vi "Stage v4.vi"() -> ()   [LabVIEW 2025]
uses:
  upper limit.ctl
  lower limit.ctl
  libximc.lvlib
panel:
  in  "Help":bool
  in  "Shift Stage Page":bool
  in  "Move to Destination Page":bool
  in  "Move Relative Page":bool
  in  "Initialize Page":bool
  in  "Tab Control":T1(tab)=enum."Shift Stage"
  out "s/n 2":u32
  out "s/n 3":u32
  out "s/n 1":u32
  in  "Controller 1":u16(ring) items=["xi-com:\\\\.\\COM3", "xi-com:\\\\.\\COM4", "xi-com:\\\\.\\COM5"]
  in  "Controller 2":u16(ring) items=["xi-com:\\\\.\\COM3", "xi-com:\\\\.\\COM4", "xi-com:\\\\.\\COM5"]
  in  "Controller 3":u16(ring) items=["xi-com:\\\\.\\COM3", "xi-com:\\\\.\\COM4", "xi-com:\\\\.\\COM5"]
  in  "Move To Destination":bool
  in  "Destination X":dbl format="%#.3f"
  in  "Destination Z":dbl format="%#.3f"
  in  "Destination Y":dbl format="%#.3f"
  in  "Update Position":bool
  in  "Paste Positions":bool
  in  "Shift X":dbl format="%#.3f"
  in  "Shift Z":dbl format="%#.3f"
  in  "Shift Y":dbl format="%#.3f"
  in  "Move Relative":bool
  in  "shift stage":bool
  in  "Shift Amount (mm)":dbl format="%#.3f"
  in  "Copy Positions":bool
  in  "Zero":bool
  in  "Go Home":bool
  in  "Exit":bool
  out "Cursor Z":dbl format="%.3f"
  out "Cursor Y":dbl format="%.3f"
  out "Cursor X":dbl format="%.3f"
  # "Controller IDs"
  # "Serial Numbers"
  # "Controller Y"
  # "Controller X"
  # "Controller Z"
  # "If serial numbers are 0, click the help button!"
  # "NOTE: Units of all positions are in mm."
  # "Stage not moving:"
  # "Check if the serial numbers are zero. If so, close this app and load the controllers in order (1, 2, then 3) in XILab. Close XILab and open this app. and controllers should load correctly."
  # "Controllers not found in XILab:"
  # "Unplug and replug USBs connecting the motors to the computer, then follow previous instructions."
  # "If you have any other questions, feel free to reach out to Erykah at erykahfoss@u.boisestate.edu"
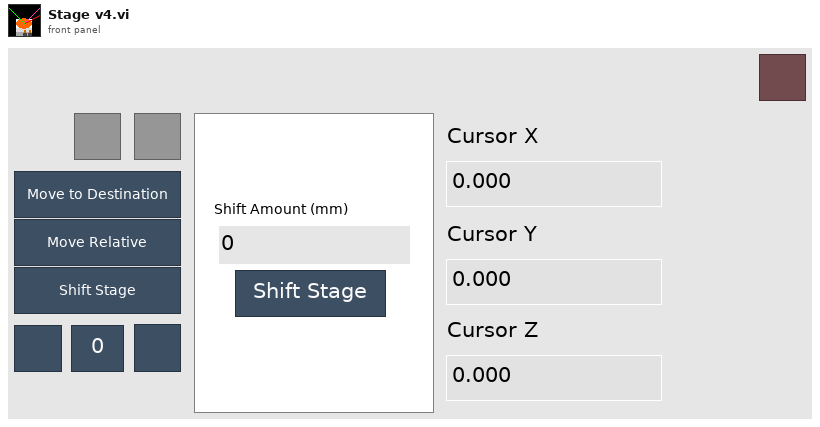
[diagram p1: front panel]
types:
  T1 = enum32{"Initialize", "Help", "Move to Destination", "Move Relative", "Shift Stage"}
  T2 = enum16{"Initialize", "Help", "Move to Destination", "Move Relative", "Shift Stage"}
  T3 = enum32{"invalid app kind", "Development System", "Run Time System", "Student Edition", "Embedded LabVIEW", "Evaluation", "Custom"}
  T4 = cluster{"Number of controllers":i32, "Controllers' names":string[], "variant":variant, "quit":bool, "IDs":i32[]}
  T5 = typedef "eventvkey.ctl" = enum16{"ASCII", "Enter", "Return", "Shift", "Ctrl", "Alt", "Cmd", "Opt", "Caps", "NumLock", "Clear", "Break", "Up", "Down", "Left", "Right", "Insert", "Delete", "Home", "End", "PageUp", "PageDown", "Escape", "Help", "Pause", "ScrollLock", "F1", "F2", "F3", "F4", "F5", "F6", "F7", "F8", "F9", "F10", "F11", "F12", "F13", "F14", "F15", "F16", "F17", "F18", "F19", "F20", "F21", "F22", "F23", "F24", "Play", "VolumeUp", "VolumeDown", "Mute", "Two Byte Char"}
  T6 = typedef "lower limit.ctl" = i32
  T7 = typedef "upper limit.ctl" = i32
  T8 = cluster{"MoveSts":u32, "MvCmdSts":u32, "PWRSts":u32, "EncSts":u32, "WindSts":u32, "CurPosition":i32, "uCurPosition":i32, "@dummy control@":i8, "@dummy control@":i8, "@dummy control@":i8, "@dummy control@":i8, "EncPosition":i64, "CurSpeed":i32, "uCurSpeed":i32, "Ipwr":i32, "Upwr":i32, "Iusb":i32, "Uusb":i32, "CurT":i32, "Flags":u32, "GPIOFlags":u32, "CmdBufFreeSpace":u32}
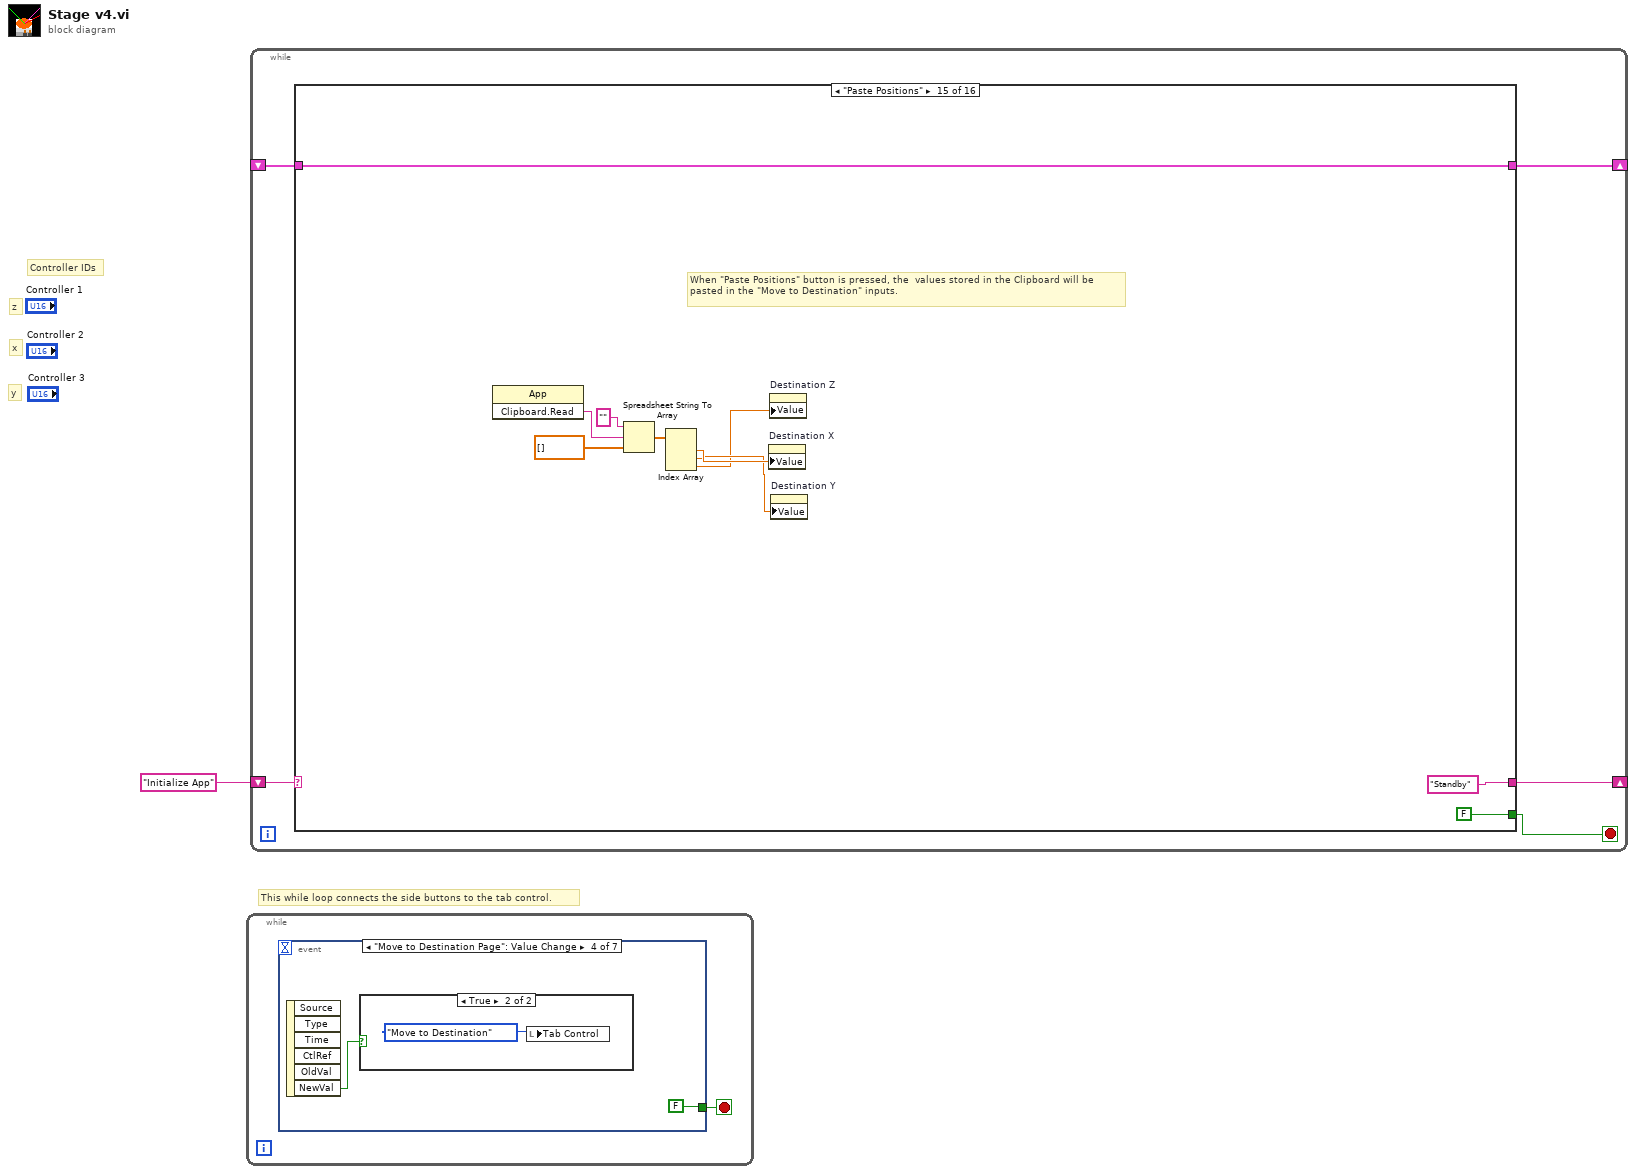
[diagram p0: block diagram]
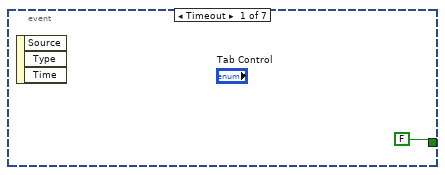
[diagram p2: hidden frame]
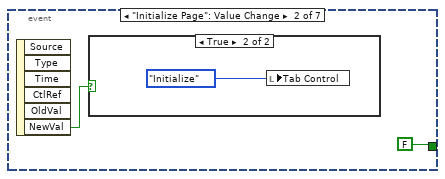
[diagram p3: hidden frame]
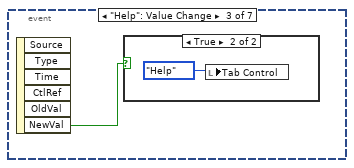
[diagram p5: hidden frame]
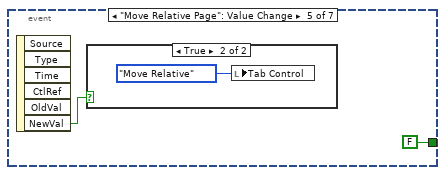
[diagram p8: hidden frame]
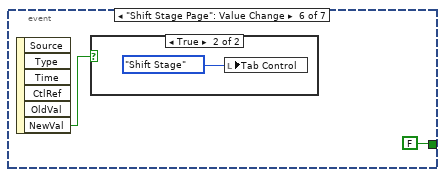
[diagram p10: hidden frame]
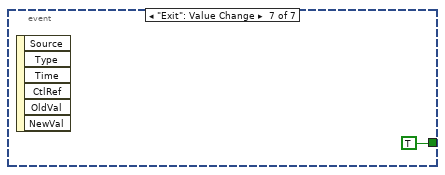
[diagram p12: hidden frame]
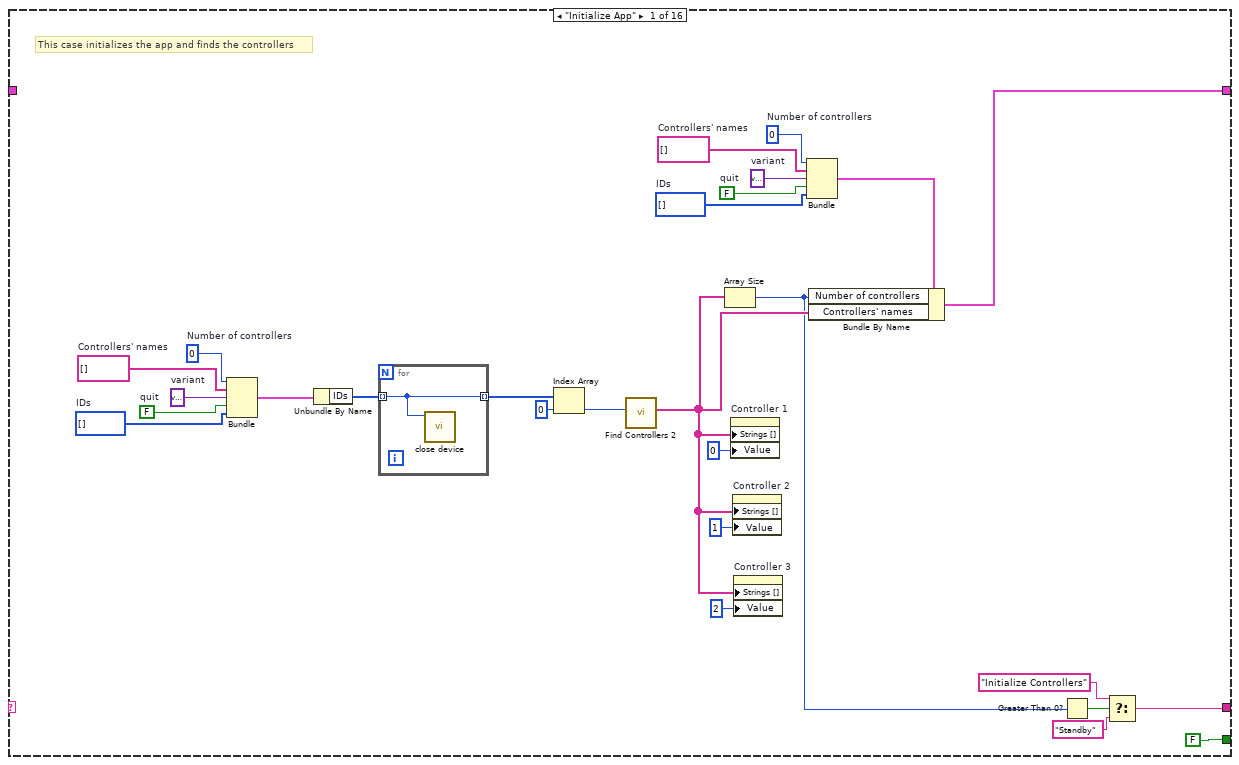
[diagram p13: hidden frame]
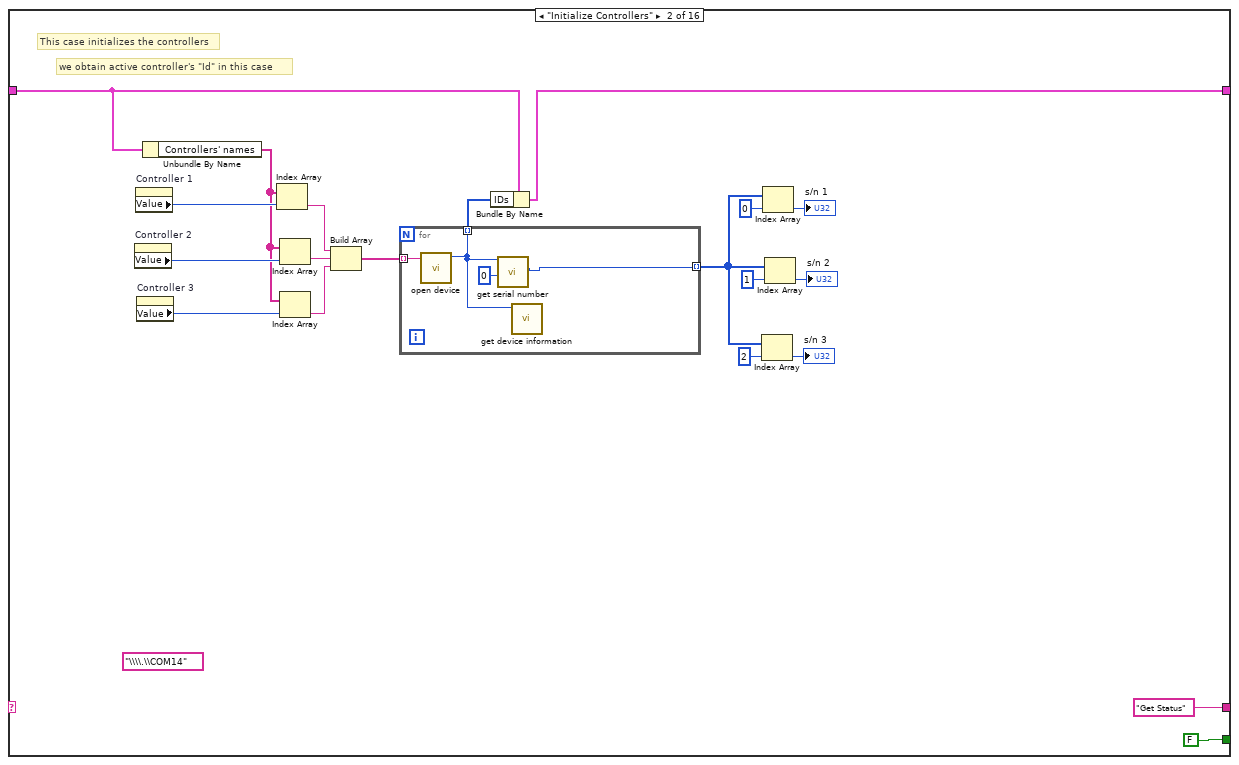
[diagram p14: hidden frame]
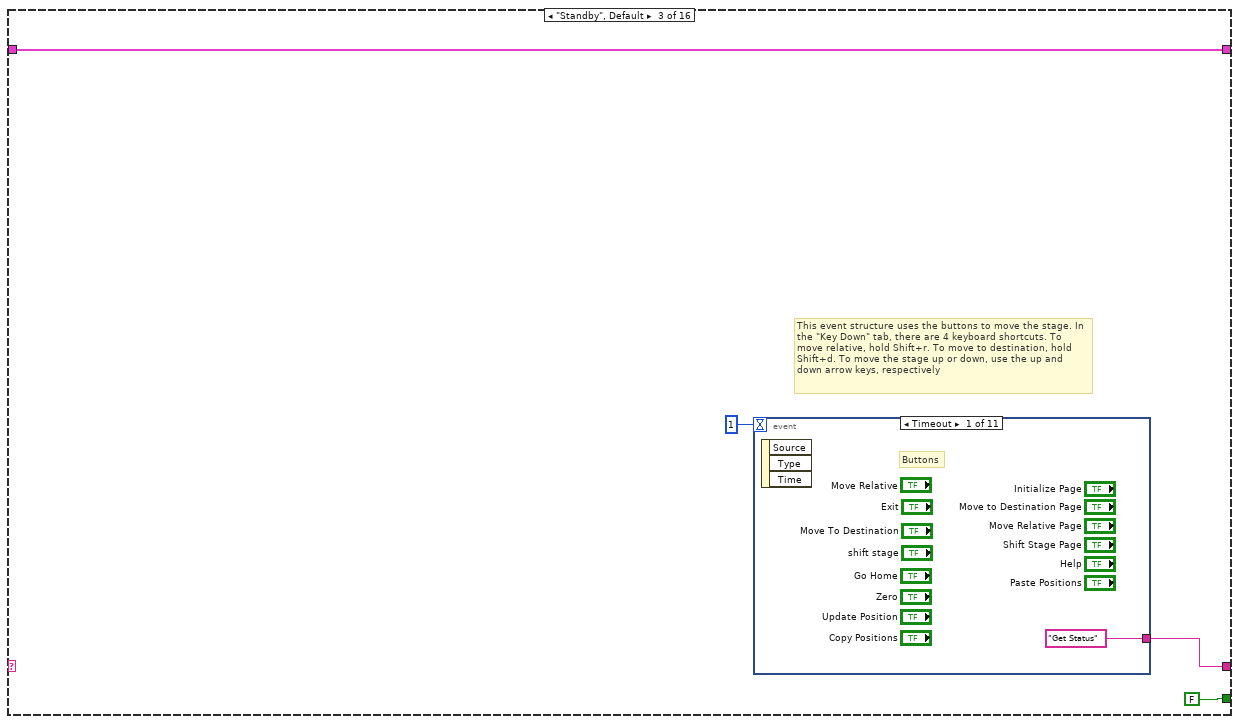
[diagram p15: hidden frame]
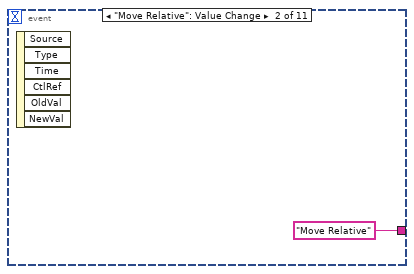
[diagram p16: hidden frame]
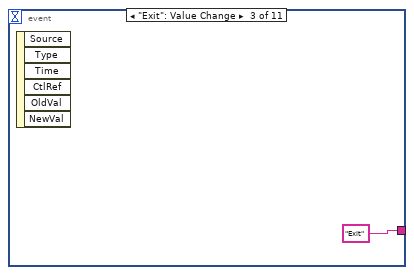
[diagram p17: hidden frame]
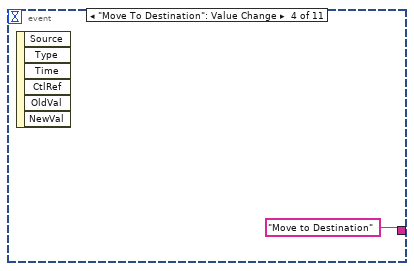
[diagram p18: hidden frame]
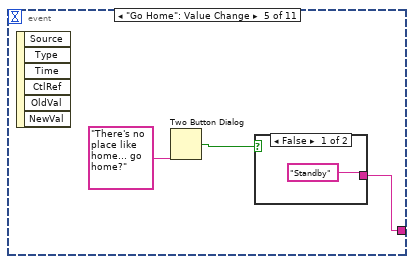
[diagram p19: hidden frame]
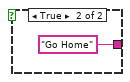
[diagram p20: hidden frame]
diagram:
  # "y"
  # "x"
  # "z"
  # "This while loop connects the side buttons to the tab control."
  # "Controller IDs"
  n1 = while {
    stop <- w2 stop-if-true
    n2 = event shown="[3] \"Move to Destination Page\": Value Change" {
      selector: _ -> [_ _ _ _ _ _ _]
      dyn-events: _ -> [_ _ _ _ _ _ _]
      timeout: _ -> [_ _ _ _ _ _ _]
      tunnel: [FALSE FALSE _ FALSE FALSE FALSE TRUE] -> w2
      event Timeout {
        n3 = event-data() -> ()  [unwired: 1 in, 3 out]
      }
      event "Initialize Page": Value Change {
        n4 = event-data() -> ("NewVal"=w4:bool)  [unwired: 1 in, 5 out]
        n5 = case shown="True" w4 {
          frame False {
          }
          frame True {
            n6 = local write "Tab Control"(T2."Initialize") -> ()
          }
        }
      }
      event "Help": Value Change {
        n7 = event-data() -> ("NewVal"=w7:bool)  [unwired: 1 in, 5 out]
        n8 = case shown="True" w7 {
          frame False {
          }
          frame True {
            n9 = local write "Tab Control"(T2."Help") -> ()
          }
        }
      }
      event "Move to Destination Page": Value Change {
        n10 = event-data() -> ("NewVal"=w9:bool)  [unwired: 1 in, 5 out]
        n11 = case shown="True" w9 {
          frame False {
          }
          frame True {
            n12 = local write "Tab Control"(T2."Move to Destination") -> ()
          }
        }
      }
      event "Move Relative Page": Value Change {
        n13 = event-data() -> ("NewVal"=w12:bool)  [unwired: 1 in, 5 out]
        n14 = case shown="True" w12 {
          frame False {
          }
          frame True {
            n15 = local write "Tab Control"(T2."Move Relative") -> ()
          }
        }
      }
      event "Shift Stage Page": Value Change {
        n16 = event-data() -> ("NewVal"=w15:bool)  [unwired: 1 in, 5 out]
        n17 = case shown="True" w15 {
          frame False {
          }
          frame True {
            n18 = local write "Tab Control"(T2."Shift Stage") -> ()
          }
        }
      }
      event "Exit": Value Change {
        n19 = event-data() -> ()  [unwired: 1 in, 6 out]
      }
    }
  }
  n20 = while {
    shift-right: [w22] -> _
    shift-left: _ -> [w23]
    shift-right: [w21] -> _
    shift-left: "Initialize App" -> [w20]
    stop <- w19 stop-if-true
    n21 = case shown="\"Paste Positions\"" w20 {
      tunnel: [w44 w61 w79 w125 w175 w240 w292 w349 w411 w460 w465 w470 w482 w504 w514 w522] -> w22
      tunnel: w23 -> [_ w62 w79 w125 w175 w239 w292 w349 w411 w460 w465 w470 w482 w504 w514 w522]
      tunnel: [w25 "Get Status" w77 w138 w174 w238 w291 w348 w410 "Standby" "Standby" "Standby" "Standby" "Standby" "Standby" "Standby"] -> w21
      tunnel: [FALSE ("quit") FALSE ("quit") FALSE ("quit") w127 FALSE ("quit") FALSE ("quit") FALSE FALSE FALSE FALSE FALSE FALSE FALSE FALSE FALSE TRUE ("quit")] -> w19
      frame "Initialize App" {
        w31 = i32[] []  # IDs
        w32 = FALSE  # quit
        w33 = variant  # variant
        w34 = string[] []  # Controllers' names
        w35 = 0  # Number of controllers
        w46 = i32[] []  # IDs
        w47 = FALSE  # quit
        w48 = variant  # variant
        w49 = string[] []  # Controllers' names
        w50 = 0  # Number of controllers
        # "This case initializes the app and finds the controllers"
        n22 = Bundle("Number of controllers"=w35, "Controllers' names"=w34, "variant"=w33, "quit"=w32, "IDs"=w31) -> (w30:T4)  [unwired: 1 in]
        n23 = Unbundle By Name(w30) -> ("IDs"=w37:i32[])
        n24 = for {
          tunnel: w37 -> [w51] mode=indexing
          tunnel: [w51] -> w36 mode=indexing
          n25 = call "close device.vi"("id"=w51) -> ()  [unwired: 8 in, 3 out]
        }
        n26 = Index Array(array=w36, index=0) -> (element=w42:i32)
        n27 = call "Find Controllers 2.vi"("Numeric"=w42) -> ("Names"=w38:string[])  [unwired: 9 in, 1 out]
        n28 = Array Size(array=w38) -> (size(s)=w28:i32)
        n29 = property on="Controller 1" class="Ring (strict)"("Strings []"=w38, "Value"=0) -> ()  [unwired: 2 in, 2 out]
        n30 = property on="Controller 2" class="Ring (strict)"("Strings []"=w38, "Value"=1) -> ()  [unwired: 2 in, 2 out]
        n31 = property on="Controller 3" class="Ring (strict)"("Strings []"=w38, "Value"=2 ("Controller 3")) -> ()  [unwired: 2 in, 2 out]
        n32 = Bundle("Number of controllers"=w50, "Controllers' names"=w49, "variant"=w48, "quit"=w47, "IDs"=w46) -> (w45:T4)  [unwired: 1 in]
        n33 = Bundle By Name(cluster=w45, "Number of controllers"=w28, "Controllers' names"=w38) -> (w44:T4)
        n34 = Greater Than 0?(x=w28) -> (x > 0?=w29:bool)
        n35 = Select(t="Initialize Controllers", s=w29, f="Standby") -> (s? t:f=w25:string)
      }
      frame "Initialize Controllers" {
        (unwired) "\\\\.\\COM14" ("name")
        # "we obtain active controller's \"Id\" in this case"
        # "This case initializes the controllers"
        n36 = property on="Controller 2" class="Ring (strict)"() -> ("Value"=w70:u16)  [unwired: 2 in, 2 out]
        n37 = property on="Controller 1" class="Ring (strict)"() -> ("Value"=w71:u16)  [unwired: 2 in, 2 out]
        n38 = property on="Controller 3" class="Ring (strict)"() -> ("Value"=w69:u16)  [unwired: 2 in, 2 out]
        n39 = Unbundle By Name(w62) -> ("Controllers' names"=w65:string[])
        n40 = Index Array(array=w65, index=w71) -> (element=w66:string)
        n41 = Index Array(array=w65, index=w70) -> (element=w67:string)
        n42 = Index Array(array=w65, index=w69) -> (element=w68:string)
        n43 = Build Array(w66, w67, w68) -> (w64:string[])
        n44 = for {
          tunnel: w64 -> [w75] mode=indexing
          tunnel: [w73] -> w63 mode=indexing
          tunnel: [w72] -> w54 mode=indexing
          n45 = call "open device.vi"("uri"=w75) -> ("function return"=w73:i32)  [unwired: 9 in, 1 out]
          n46 = call "get serial number.vi"("SerialNumber"=0, "id"=w73) -> ("SerialNumber out"=w72:u32)  [unwired: 7 in, 2 out]
          n47 = call "get device information.vi"("id"=w73) -> ()  [unwired: 8 in, 3 out]
        }
        n48 = Bundle By Name(cluster=w62, "IDs"=w63) -> (w61:T4)
        n49 = Index Array(array=w54, index=u32 2 ("serial")) -> (element=→"s/n 3":u32)
        n50 = Index Array(array=w54, index=u32 0 ("serial")) -> (element=→"s/n 1":u32)
        n51 = Index Array(array=w54, index=u32 1 ("serial")) -> (element=→"s/n 2":u32)
      }
      frame "Standby", Default {
        # "This event structure uses the buttons to move the stage. In the \"Key Down\" tab, there are 4 keyboard shortcuts. To move relative, hold Shift+r. To move to destination, hold Shift+d. To move the stage up or down, use the up and down arrow keys, respectively"
        n52 = event shown="[0] Timeout" {
          selector: _ -> [_ _ _ _ _ _ _ _ _ _ _]
          dyn-events: _ -> [_ _ _ _ _ _ _ _ _ _ _]
          timeout: 1 -> [_ _ _ _ _ _ _ _ _ _ _]
          tunnel: ["Get Status" "Move Relative" "Exit" "Move to Destination" w86 w91 "Shift Stage" "Update Position" "Copy Positions" "Paste Positions" w100] -> w77
          event Timeout {
            # "Buttons"
            n53 = event-data() -> ()  [unwired: 1 in, 3 out]
          }
          event "Move Relative": Value Change {
            n54 = event-data() -> ()  [unwired: 1 in, 6 out]
          }
          event "Exit": Value Change {
            n55 = event-data() -> ()  [unwired: 1 in, 6 out]
          }
          event "Move To Destination": Value Change {
            n56 = event-data() -> ()  [unwired: 1 in, 6 out]
          }
          event "Go Home": Value Change {
            n57 = event-data() -> ()  [unwired: 1 in, 6 out]
            n58 = Two Button Dialog(message="There's no place like home... go home?") -> (T button?=w85:bool)  [unwired: 2 in]
            n59 = case shown="False" w85 {
              tunnel: ["Standby" "Go Home"] -> w86
              frame False {
              }
              frame True {
              }
            }
          }
          event "Zero": Value Change {
            n60 = event-data() -> ()  [unwired: 1 in, 6 out]
            n61 = Two Button Dialog(message="Zero stage?") -> (T button?=w89:bool)  [unwired: 2 in]
            n62 = case shown="False" w89 {
              tunnel: ["Standby" "Zero"] -> w91
              frame False {
              }
              frame True {
              }
            }
          }
          event "shift stage": Value Change {
            n63 = event-data() -> ()  [unwired: 1 in, 6 out]
          }
          event "Update Position": Value Change {
            n64 = event-data() -> ()  [unwired: 1 in, 6 out]
          }
          event "Copy Positions": Value Change {
            n65 = event-data() -> ()  [unwired: 1 in, 6 out]
          }
          event "Paste Positions": Value Change {
            n66 = event-data() -> ()  [unwired: 1 in, 6 out]
          }
          event Key Down {
            n67 = event-data() -> ("Char"=w99:i16, "VKey"=w98:T5)  [unwired: 1 in]
            n68 = case shown="0, Default" w99 {
              tunnel: [w101 "Move Relative" "Move to Destination" "Standby" "Standby"] -> w100
              tunnel: w98 -> [w102 _ _ _ _]
              frame 0, Default {
                n69 = case shown="\"ASCII\", Default" w102 {
                  tunnel: ["Get Status" "Shift Up" "Shift Down"] -> w101
                  frame "ASCII", Default {
                  }
                  frame "Up" {
                  }
                  frame "Down" {
                  }
                }
              }
              frame 82 {
              }
              frame 68 {
              }
              frame 102 {
                n70 = call <vilib>:"Application Directory.vi"() -> ("Application Directory"=w111:path)
                n71 = String To Path(string="f.wav") -> (path=w109:path)
                n72 = Build Path(base path=w111, name or relative path=w109) -> (appended path=w108:path)
                n73 = call <vilib>:"Play Sound File.vi"("path"=w108) -> ()  [unwired: 9 in, 2 out]
              }
              frame 108 {
                n74 = call <vilib>:"Application Directory.vi"() -> ("Application Directory"=w116:path)
                n75 = String To Path(string="l.wav") -> (path=w114:path)
                n76 = Build Path(base path=w116, name or relative path=w114) -> (appended path=w113:path)
                n77 = call <vilib>:"Play Sound File.vi"("path"=w113) -> ()  [unwired: 9 in, 2 out]
              }
            }
          }
        }
      }
      frame "Get Status" {
        w123 = 8.3e-05
        w126 = T6 -600
        w128 = T7 156626
        # "step to mm"
        # "cursor 3"
        # "cursor 2"
        # "cursor 1"
        # "lower limit"
        # "upper limit"
        # "Note: The upper limit comes from a calculation. The motor upper limit is 13 mm, and a step size is 0.083 um (https://www.standa.lt/products/catalog/motorised_positioners?item=315). The conversion is then 13 mm = 156,626 steps. Assuming that the motors are zeroed at the lowest height, the lower limit would be 0 mm = 0 steps and the upper limit would be 13 mm = 156,626 steps.\n\nMotors can't be zeroed in this LabVIEW program... this would be a good thing to include."
        # "These \"OR\" statements should check if any of the motors are at or above their upper limits or at or below thier lower limits."
        n78 = Unbundle By Name(w125) -> ("IDs"=w147:i32[])
        n79 = for {
          tunnel: [w161] -> w145 mode=indexing
          tunnel: w147 -> [w160] mode=indexing
          tunnel: [w159] -> w146 mode=indexing
          n80 = call "get status.vi"("id"=w160) -> ("status out"=w158:T8, "function return"=w159:i32)  [unwired: 8 in, 1 out]
          n81 = Unbundle By Name(w158) -> ("CurPosition"=w161:i32)
        }
        n82 = Greater Or Equal To 0?(x=w146) -> (x >= 0?=w141:bool[])
        n83 = And Array Elements(Boolean array=w141) -> ()  [unwired: 1 out]
        n84 = Index Array(array=w145, index #1=0 ("index"), index #2=1 ("index"), index #3=2 ("index")) -> (element #1=w124:i32, element #2=w122:i32, element #3=w121:i32)
        n85 = Less?(x=w124, y=w126) -> (x < y?=w139:bool)
        n86 = Greater Or Equal?(x=w124, y=w128) -> (x >= y?=w140:bool)
        n87 = Multiply(x=w123, y=w124) -> (x*y=→"Cursor Z":dbl)
        n88 = Multiply(x=w123, y=w122) -> (x*y=→"Cursor X":dbl)
        n89 = Multiply(x=w123, y=w121) -> (x*y=→"Cursor Y":dbl)
        n90 = Or(x=w140, y=w139) -> (x .or. y?=w133:bool)
        n91 = Greater Or Equal?(x=w122, y=w128) -> (x >= y?=w137:bool)
        n92 = Less?(x=w122, y=w126) -> (x < y?=w136:bool)
        n93 = Or(x=w137, y=w136) -> (x .or. y?=w132:bool)
        n94 = Greater Or Equal?(x=w121, y=w128) -> (x >= y?=w135:bool)
        n95 = Less?(x=w121, y=w126) -> (x < y?=w134:bool)
        n96 = Or(x=w135, y=w134) -> (x .or. y?=w131:bool)
        n97 = Build Array(w133, w132, w131) -> (w130:bool[])
        n98 = Or Array Elements(Boolean array=w130) -> (logical OR=w129:bool)
        n99 = case shown="False" w129 {
          tunnel: ["Standby" "Stop Motion"] -> w138
          tunnel: [FALSE w155] -> w127
          frame False {
          }
          frame True {
            # "If any of them move past the limits, the program will stop. You won't be able to use this LabVIEW program until the height is fixed in XILab."
            n100 = call <vilib>:"Application Directory.vi"() -> ("Application Directory"=w154:path)
            n101 = String To Path(string="l.wav") -> (path=w152:path)
            n102 = Build Path(base path=w154, name or relative path=w152) -> (appended path=w151:path)
            n103 = call <vilib>:"Sound File Read Simple.vi"("path"=w151) -> ("path out"=w150:path)  [unwired: 7 in, 3 out]
            n104 = call <vilib>:"Play Sound File.vi"("path"=w150) -> ()  [unwired: 9 in, 2 out]
            n105 = One Button Dialog(message="You've gone too far this time...\nPlease check the height of the stage and move it back to a normal height using XILab <3") -> (true=w155:bool)  [unwired: 1 in]
          }
        }
      }
      frame "Move Relative" {
        w171 = 8.3e-05
        w172 = T7 156626
        w173 = -1
        # "mm to step"
        # "in mm"
        # "cursor 3"
        # "cursor 2"
        # "cursor 1"
        # "lower limit"
        # "upper limit"
        n106 = Unbundle By Name(w175) -> ("IDs"=w199:i32[])
        n107 = for {
          tunnel: [w225] -> w197 mode=indexing
          tunnel: w199 -> [w224] mode=indexing
          tunnel: [w223] -> w198 mode=indexing
          n108 = call "get status.vi"("id"=w224) -> ("status out"=w222:T8, "function return"=w223:i32)  [unwired: 8 in, 1 out]
          n109 = Unbundle By Name(w222) -> ("CurPosition"=w225:i32)
        }
        n110 = Greater Or Equal To 0?(x=w198) -> (x >= 0?=w193:bool[])
        n111 = And Array Elements(Boolean array=w193) -> ()  [unwired: 1 out]
        n112 = Index Array(array=w197, index #1=0 ("index"), index #2=1 ("index"), index #3=2 ("index")) -> (element #1=w181:i32, element #2=w180:i32, element #3=w179:i32)
        n113 = Divide(x="Shift Y", y=w171) -> (x/y=w167:dbl)
        n114 = Divide(x="Shift Z", y=w171) -> (x/y=w165:dbl)
        n115 = Divide(x="Shift X", y=w171) -> (x/y=w163:dbl)
        n116 = To Long Integer(number=w167) -> (32bit integer=w166:i32)
        n117 = To Long Integer(number=w165) -> (32bit integer=w164:i32)
        n118 = Add(x=w166, y=w181) -> (x+y=w178:i32)
        n119 = Add(x=w164, y=w180) -> (x+y=w176:i32)
        n120 = To Long Integer(number=w163) -> (32bit integer=w162:i32)
        n121 = Add(x=w162, y=w179) -> (x+y=w177:i32)
        n122 = Less Or Equal?(x=w178, y=w173) -> (x <= y?=w191:bool)
        n123 = Greater Or Equal?(x=w177, y=w172) -> (x >= y?=w188:bool)
        n124 = Greater Or Equal?(x=w178, y=w172) -> (x >= y?=w192:bool)
        n125 = Greater Or Equal?(x=w176, y=w172) -> (x >= y?=w190:bool)
        n126 = Less Or Equal?(x=w176, y=w173) -> (x <= y?=w189:bool)
        n127 = Less Or Equal?(x=w177, y=w173) -> (x <= y?=w187:bool)
        n128 = Or(x=w188, y=w187) -> (x .or. y?=w184:bool)
        n129 = Or(x=w190, y=w189) -> (x .or. y?=w185:bool)
        n130 = Or(x=w192, y=w191) -> (x .or. y?=w186:bool)
        n131 = Build Array(w186, w185, w184) -> (w183:bool[])
        n132 = Or Array Elements(Boolean array=w183) -> (logical OR=w182:bool)
        n133 = case shown="False" w182 {
          tunnel: ["Standby" "Stop Motion"] -> w174
          tunnel: w175 -> [w211 w219]
          tunnel: [w209 w219] -> _
          tunnel: w166 -> [w203 _]
          tunnel: w164 -> [w202 _]
          tunnel: w162 -> [w201 _]
          frame False {
            n134 = Bundle(w202, w201, w203) -> (w210:cluster{i32, i32, i32})  [unwired: 1 in]
            n135 = Bundle By Name(cluster=w211, "variant"=w210) -> (w209:T4)
            n136 = Unbundle By Name(w209) -> ("IDs"=w204:i32[], "variant"=w206:variant)
            n137 = Variant To Data(type=cluster{u32, u32, u32} {0, 0, 0}, Variant=w206) -> (data=w207:cluster{u32, u32, u32})  [unwired: 1 in, 1 out]
            n138 = Cluster To Array(cluster=w207) -> (array=w208:u32[])
            n139 = for {
              tunnel: w208 -> [w213] mode=indexing
              tunnel: w204 -> [w214] mode=indexing
              n140 = call "command movr.vi"("DeltaPosition"=w213, "id"=w214) -> ()  [unwired: 8 in, 2 out]
            }
          }
          frame True {
            # "If any of them move past the limits, the motors won't move."
            n141 = call <vilib>:"Application Directory.vi"() -> ("Application Directory"=w218:path)
            n142 = String To Path(string="l.wav") -> (path=w216:path)
            n143 = Build Path(base path=w218, name or relative path=w216) -> (appended path=w215:path)
            n144 = One Button Dialog(message="You've gone too far this time...\nPlease ensure the step size does not go past the limits <3") -> ()  [unwired: 1 in, 1 out]
            n145 = call <vilib>:"Play Sound File.vi"("path"=w215) -> ()  [unwired: 9 in, 2 out]
          }
        }
      }
      frame "Move to Destination" {
        w232 = 8.3e-05
        w236 = T7 156626
        w237 = -1
        # "mm to step"
        # "cursor 3"
        # "cursor 2"
        # "cursor 1"
        # "lower limit"
        # "upper limit"
        n146 = Unbundle By Name(w239) -> ("IDs"=w258:i32[])
        n147 = for {
          tunnel: [w284] -> w256 mode=indexing
          tunnel: w258 -> [w283] mode=indexing
          tunnel: [w282] -> w257 mode=indexing
          n148 = call "get status.vi"("id"=w283) -> ("status out"=w281:T8, "function return"=w282:i32)  [unwired: 8 in, 1 out]
          n149 = Unbundle By Name(w281) -> ("CurPosition"=w284:i32)
        }
        n150 = Greater Or Equal To 0?(x=w257) -> (x >= 0?=w252:bool[])
        n151 = And Array Elements(Boolean array=w252) -> ()  [unwired: 1 out]
        n152 = Index Array(array=w256, index #1=0 ("index"), index #2=1 ("index"), index #3=2 ("index")) -> ()  [unwired: 3 out]
        n153 = Divide(x="Destination Y", y=w232) -> (x/y=w231:dbl)
        n154 = Divide(x="Destination Z", y=w232) -> (x/y=w229:dbl)
        n155 = Divide(x="Destination X", y=w232) -> (x/y=w227:dbl)
        n156 = To Long Integer(number=w231) -> (32bit integer=w230:i32)
        n157 = To Long Integer(number=w227) -> (32bit integer=w226:i32)
        n158 = To Long Integer(number=w229) -> (32bit integer=w228:i32)
        n159 = Less Or Equal?(x=w230, y=w237) -> (x <= y?=w250:bool)
        n160 = Greater Or Equal?(x=w226, y=w236) -> (x >= y?=w247:bool)
        n161 = Greater Or Equal?(x=w230, y=w236) -> (x >= y?=w251:bool)
        n162 = Greater Or Equal?(x=w228, y=w236) -> (x >= y?=w249:bool)
        n163 = Less Or Equal?(x=w228, y=w237) -> (x <= y?=w248:bool)
        n164 = Less Or Equal?(x=w226, y=w237) -> (x <= y?=w246:bool)
        n165 = Or(x=w247, y=w246) -> (x .or. y?=w243:bool)
        n166 = Or(x=w249, y=w248) -> (x .or. y?=w244:bool)
        n167 = Or(x=w251, y=w250) -> (x .or. y?=w245:bool)
        n168 = Build Array(w245, w244, w243) -> (w242:bool[])
        n169 = Or Array Elements(Boolean array=w242) -> (logical OR=w241:bool)
        n170 = case shown="False" w241 {
          tunnel: ["Standby" "Stop Motion"] -> w238
          tunnel: w239 -> [w264 w278]
          tunnel: [w263 w278] -> w240
          tunnel: w230 -> [w261 _]
          tunnel: w228 -> [w260 _]
          tunnel: w226 -> [w262 _]
          frame False {
            n171 = Bundle(w260, w262, w261) -> (w266:cluster{i32, i32, i32})  [unwired: 1 in]
            n172 = Bundle By Name(cluster=w264, "variant"=w266) -> (w263:T4)
            n173 = Unbundle By Name(w263) -> ("IDs"=w268:i32[], "variant"=w270:variant)
            n174 = Variant To Data(type=cluster{u32, u32, u32} {0, 0, 0}, Variant=w270) -> (data=w267:cluster{u32, u32, u32})  [unwired: 1 in, 1 out]
            n175 = Cluster To Array(cluster=w267) -> (array=w269:u32[])
            n176 = for {
              tunnel: w269 -> [w272] mode=indexing
              tunnel: w268 -> [w273] mode=indexing
              n177 = call "command move.vi"("Position"=w272, "id"=w273) -> ()  [unwired: 8 in, 2 out]
            }
          }
          frame True {
            # "If any of them move past the limits, the motors won't move."
            n178 = call <vilib>:"Application Directory.vi"() -> ("Application Directory"=w277:path)
            n179 = String To Path(string="l.wav") -> (path=w275:path)
            n180 = Build Path(base path=w277, name or relative path=w275) -> (appended path=w274:path)
            n181 = call <vilib>:"Play Sound File.vi"("path"=w274) -> ()  [unwired: 9 in, 2 out]
            n182 = One Button Dialog(message="You've gone too far this time...\nPlease ensure the step size does not go past the limits <3") -> ()  [unwired: 1 in, 1 out]
          }
        }
      }
      frame "Shift Stage" {
        w289 = T7 156626
        w290 = -1
        # "mm to step"
        # "cursor 3"
        # "cursor 2"
        # "cursor 1"
        # "lower limit"
        # "upper limit"
        n183 = Unbundle By Name(w292) -> ("IDs"=w316:i32[])
        n184 = for {
          tunnel: [w340] -> w314 mode=indexing
          tunnel: w316 -> [w339] mode=indexing
          tunnel: [w338] -> w315 mode=indexing
          n185 = call "get status.vi"("id"=w339) -> ("status out"=w337:T8, "function return"=w338:i32)  [unwired: 8 in, 1 out]
          n186 = Unbundle By Name(w337) -> ("CurPosition"=w340:i32)
        }
        n187 = Greater Or Equal To 0?(x=w315) -> (x >= 0?=w310:bool[])
        n188 = And Array Elements(Boolean array=w310) -> ()  [unwired: 1 out]
        n189 = Index Array(array=w314, index #1=0 ("index"), index #2=1 ("index"), index #3=2 ("index")) -> (element #1=w298:i32, element #2=w297:i32, element #3=w296:i32)
        n190 = Divide(x="Shift Amount (mm)", y=8.3e-05) -> (x/y=w286:dbl)
        n191 = To Long Integer(number=w286) -> (32bit integer=w285:i32)
        n192 = Add(x=w285, y=w298) -> (x+y=w295:i32)
        n193 = Add(x=w285, y=w297) -> (x+y=w293:i32)
        n194 = Add(x=w285, y=w296) -> (x+y=w294:i32)
        n195 = Less Or Equal?(x=w295, y=w290) -> (x <= y?=w308:bool)
        n196 = Greater Or Equal?(x=w294, y=w289) -> (x >= y?=w305:bool)
        n197 = Greater Or Equal?(x=w295, y=w289) -> (x >= y?=w309:bool)
        n198 = Greater Or Equal?(x=w293, y=w289) -> (x >= y?=w307:bool)
        n199 = Less Or Equal?(x=w293, y=w290) -> (x <= y?=w306:bool)
        n200 = Less Or Equal?(x=w294, y=w290) -> (x <= y?=w304:bool)
        n201 = Or(x=w305, y=w304) -> (x .or. y?=w301:bool)
        n202 = Or(x=w307, y=w306) -> (x .or. y?=w302:bool)
        n203 = Or(x=w309, y=w308) -> (x .or. y?=w303:bool)
        n204 = Build Array(w303, w302, w301) -> (w300:bool[])
        n205 = Or Array Elements(Boolean array=w300) -> (logical OR=w299:bool)
        n206 = case shown="False" w299 {
          tunnel: ["Standby" "Stop Motion"] -> w291
          tunnel: w292 -> [w326 w334]
          tunnel: [w324 w334] -> _
          tunnel: w285 -> [w318 _]
          frame False {
            n207 = Bundle(w318, w318, w318) -> (w325:cluster{i32, i32, i32})  [unwired: 1 in]
            n208 = Bundle By Name(cluster=w326, "variant"=w325) -> (w324:T4)
            n209 = Unbundle By Name(w324) -> ("IDs"=w319:i32[], "variant"=w321:variant)
            n210 = Variant To Data(type=cluster{u32, u32, u32} {0, 0, 0}, Variant=w321) -> (data=w322:cluster{u32, u32, u32})  [unwired: 1 in, 1 out]
            n211 = Cluster To Array(cluster=w322) -> (array=w323:u32[])
            n212 = for {
              tunnel: w323 -> [w328] mode=indexing
              tunnel: w319 -> [w329] mode=indexing
              n213 = call "command movr.vi"("DeltaPosition"=w328, "id"=w329) -> ()  [unwired: 8 in, 2 out]
            }
          }
          frame True {
            # "If any of them move past the limits, the motors won't move."
            n214 = call <vilib>:"Application Directory.vi"() -> ("Application Directory"=w333:path)
            n215 = String To Path(string="l.wav") -> (path=w331:path)
            n216 = Build Path(base path=w333, name or relative path=w331) -> (appended path=w330:path)
            n217 = call <vilib>:"Play Sound File.vi"("path"=w330) -> ()  [unwired: 9 in, 2 out]
            n218 = One Button Dialog(message="You've gone too far this time...\nPlease ensure the step size does not go past the limits <3") -> ()  [unwired: 1 in, 1 out]
          }
        }
      }
      frame "Shift Up" {
        w345 = T7 156626
        w346 = -1
        # "mm to step"
        # "cursor 3"
        # "cursor 2"
        # "cursor 1"
        # "lower limit"
        # "upper limit"
        n219 = Unbundle By Name(w349) -> ("IDs"=w373:i32[])
        n220 = for {
          tunnel: [w399] -> w371 mode=indexing
          tunnel: w373 -> [w398] mode=indexing
          tunnel: [w397] -> w372 mode=indexing
          n221 = call "get status.vi"("id"=w398) -> ("status out"=w396:T8, "function return"=w397:i32)  [unwired: 8 in, 1 out]
          n222 = Unbundle By Name(w396) -> ("CurPosition"=w399:i32)
        }
        n223 = Greater Or Equal To 0?(x=w372) -> (x >= 0?=w367:bool[])
        n224 = And Array Elements(Boolean array=w367) -> ()  [unwired: 1 out]
        n225 = local read "Shift Amount (mm)"() -> (w347:dbl)
        n226 = Index Array(array=w371, index #1=0 ("index"), index #2=1 ("index"), index #3=2 ("index")) -> (element #1=w355:i32, element #2=w354:i32, element #3=w353:i32)
        n227 = Absolute Value(x=w347) -> (abs(x)=w344:dbl)
        n228 = Divide(x=w344, y=8.3e-05) -> (x/y=w342:dbl)
        n229 = To Long Integer(number=w342) -> (32bit integer=w341:i32)
        n230 = Add(x=w341, y=w355) -> (x+y=w352:i32)
        n231 = Add(x=w341, y=w354) -> (x+y=w350:i32)
        n232 = Add(x=w341, y=w353) -> (x+y=w351:i32)
        n233 = Less Or Equal?(x=w352, y=w346) -> (x <= y?=w365:bool)
        n234 = Greater Or Equal?(x=w351, y=w345) -> (x >= y?=w362:bool)
        n235 = Greater Or Equal?(x=w352, y=w345) -> (x >= y?=w366:bool)
        n236 = Greater Or Equal?(x=w350, y=w345) -> (x >= y?=w364:bool)
        n237 = Less Or Equal?(x=w350, y=w346) -> (x <= y?=w363:bool)
        n238 = Less Or Equal?(x=w351, y=w346) -> (x <= y?=w361:bool)
        n239 = Or(x=w362, y=w361) -> (x .or. y?=w358:bool)
        n240 = Or(x=w364, y=w363) -> (x .or. y?=w359:bool)
        n241 = Or(x=w366, y=w365) -> (x .or. y?=w360:bool)
        n242 = Build Array(w360, w359, w358) -> (w357:bool[])
        n243 = Or Array Elements(Boolean array=w357) -> (logical OR=w356:bool)
        n244 = case shown="False" w356 {
          tunnel: ["Standby" "Stop Motion"] -> w348
          tunnel: w341 -> [w385 _]
          tunnel: w341 -> [w384 _]
          tunnel: w341 -> [w383 _]
          tunnel: w349 -> [w382 w393]
          tunnel: [w380 w393] -> _
          frame False {
            n245 = Bundle(w385, w384, w383) -> (w381:cluster{i32, i32, i32})  [unwired: 1 in]
            n246 = Bundle By Name(cluster=w382, "variant"=w381) -> (w380:T4)
            n247 = Unbundle By Name(w380) -> ("IDs"=w375:i32[], "variant"=w377:variant)
            n248 = Variant To Data(type=cluster{u32, u32, u32} {0, 0, 0}, Variant=w377) -> (data=w378:cluster{u32, u32, u32})  [unwired: 1 in, 1 out]
            n249 = Cluster To Array(cluster=w378) -> (array=w379:u32[])
            n250 = for {
              tunnel: w379 -> [w387] mode=indexing
              tunnel: w375 -> [w388] mode=indexing
              n251 = call "command movr.vi"("DeltaPosition"=w387, "id"=w388) -> ()  [unwired: 8 in, 2 out]
            }
          }
          frame True {
            # "If any of them move past the limits, the motors won't move."
            n252 = call <vilib>:"Application Directory.vi"() -> ("Application Directory"=w392:path)
            n253 = String To Path(string="l.wav") -> (path=w390:path)
            n254 = Build Path(base path=w392, name or relative path=w390) -> (appended path=w389:path)
            n255 = call <vilib>:"Play Sound File.vi"("path"=w389) -> ()  [unwired: 9 in, 2 out]
            n256 = One Button Dialog(message="You've gone too far this time...\nPlease ensure the step size does not go past the limits <3") -> ()  [unwired: 1 in, 1 out]
          }
        }
      }
      frame "Shift Down" {
        w404 = T7 156626
        w413 = -1
        # "mm to step"
        # "cursor 3"
        # "cursor 2"
        # "cursor 1"
        # "lower limit"
        # "upper limit"
        n257 = Unbundle By Name(w411) -> ("IDs"=w433:i32[])
        n258 = for {
          tunnel: [w459] -> w431 mode=indexing
          tunnel: w433 -> [w458] mode=indexing
          tunnel: [w457] -> w432 mode=indexing
          n259 = call "get status.vi"("id"=w458) -> ("status out"=w456:T8, "function return"=w457:i32)  [unwired: 8 in, 1 out]
          n260 = Unbundle By Name(w456) -> ("CurPosition"=w459:i32)
        }
        n261 = Greater Or Equal To 0?(x=w432) -> (x >= 0?=w427:bool[])
        n262 = And Array Elements(Boolean array=w427) -> ()  [unwired: 1 out]
        n263 = local read "Shift Amount (mm)"() -> (w409:dbl)
        n264 = Index Array(array=w431, index #1=0 ("index"), index #2=1 ("index"), index #3=2 ("index")) -> (element #1=w408:i32, element #2=w407:i32, element #3=w406:i32)
        n265 = Absolute Value(x=w409) -> (abs(x)=w402:dbl)
        n266 = Divide(x=w402, y=8.3e-05) -> (x/y=w401:dbl)
        n267 = To Long Integer(number=w401) -> (32bit integer=w400:i32)
        n268 = Subtract(x=w408, y=w400) -> (x-y=w415:i32)
        n269 = Subtract(x=w407, y=w400) -> (x-y=w412:i32)
        n270 = Subtract(x=w406, y=w400) -> (x-y=w414:i32)
        n271 = Less Or Equal?(x=w415, y=w413) -> (x <= y?=w425:bool)
        n272 = Greater Or Equal?(x=w414, y=w404) -> (x >= y?=w422:bool)
        n273 = Greater Or Equal?(x=w415, y=w404) -> (x >= y?=w426:bool)
        n274 = Greater Or Equal?(x=w412, y=w404) -> (x >= y?=w424:bool)
        n275 = Less Or Equal?(x=w412, y=w413) -> (x <= y?=w423:bool)
        n276 = Less Or Equal?(x=w414, y=w413) -> (x <= y?=w421:bool)
        n277 = Or(x=w422, y=w421) -> (x .or. y?=w418:bool)
        n278 = Or(x=w424, y=w423) -> (x .or. y?=w419:bool)
        n279 = Or(x=w426, y=w425) -> (x .or. y?=w420:bool)
        n280 = Negate(x=w400) -> (-x=w405:i32)
        n281 = Build Array(w420, w419, w418) -> (w417:bool[])
        n282 = Or Array Elements(Boolean array=w417) -> (logical OR=w416:bool)
        n283 = case shown="False" w416 {
          tunnel: ["Standby" "Stop Motion"] -> w410
          tunnel: w405 -> [w445 _]
          tunnel: w405 -> [w444 _]
          tunnel: w405 -> [w443 _]
          tunnel: w411 -> [w442 w453]
          tunnel: [w440 w453] -> _
          frame False {
            n284 = Bundle(w445, w444, w443) -> (w441:cluster{i32, i32, i32})  [unwired: 1 in]
            n285 = Bundle By Name(cluster=w442, "variant"=w441) -> (w440:T4)
            n286 = Unbundle By Name(w440) -> ("IDs"=w435:i32[], "variant"=w437:variant)
            n287 = Variant To Data(type=cluster{u32, u32, u32} {0, 0, 0}, Variant=w437) -> (data=w438:cluster{u32, u32, u32})  [unwired: 1 in, 1 out]
            n288 = Cluster To Array(cluster=w438) -> (array=w439:u32[])
            n289 = for {
              tunnel: w439 -> [w447] mode=indexing
              tunnel: w435 -> [w448] mode=indexing
              n290 = call "command movr.vi"("DeltaPosition"=w447, "id"=w448) -> ()  [unwired: 8 in, 2 out]
            }
          }
          frame True {
            # "If any of them move past the limits, the motors won't move."
            n291 = call <vilib>:"Application Directory.vi"() -> ("Application Directory"=w452:path)
            n292 = String To Path(string="l.wav") -> (path=w450:path)
            n293 = Build Path(base path=w452, name or relative path=w450) -> (appended path=w449:path)
            n294 = call <vilib>:"Play Sound File.vi"("path"=w449) -> ()  [unwired: 9 in, 2 out]
            n295 = One Button Dialog(message="You've gone too far this time...\nPlease ensure the step size does not go past the limits <3") -> ()  [unwired: 1 in, 1 out]
          }
        }
      }
      frame "Stop Motion" {
        n296 = Unbundle By Name(w460) -> ("IDs"=w461:i32[])
        n297 = for {
          tunnel: w461 -> [w464] mode=indexing
          n298 = call "command stop.vi"("id"=w464) -> ()  [unwired: 9 in, 2 out]
        }
      }
      frame "Go Home" {
        n299 = Unbundle By Name(w465) -> ("IDs"=w466:i32[])
        n300 = for {
          tunnel: w466 -> [w469] mode=indexing
          n301 = call "command home.vi"("id"=w469) -> ()  [unwired: 9 in, 2 out]
        }
      }
      frame "Zero" {
        n302 = Unbundle By Name(w470) -> ("IDs"=w471:i32[])
        n303 = for {
          tunnel: w471 -> [w474] mode=indexing
          n304 = call "command zero.vi"("id"=w474) -> ()  [unwired: 9 in, 2 out]
        }
      }
      frame "Update Position" {
        w478 = 8.3e-05
        # "steps to mm"
        # "When the \"Update Position\" button is pressed, the cursor destinations in the \"Move to Destination\" tab will populate with the current cursor positions."
        n305 = Unbundle By Name(w482) -> ("IDs"=w489:i32[])
        n306 = for {
          tunnel: [w495] -> w487 mode=indexing
          tunnel: w489 -> [w494] mode=indexing
          tunnel: [w493] -> w488 mode=indexing
          n307 = call "get status.vi"("id"=w494) -> ("status out"=w492:T8, "function return"=w493:i32)  [unwired: 8 in, 1 out]
          n308 = Unbundle By Name(w492) -> ("CurPosition"=w495:i32)
        }
        n309 = Greater Or Equal To 0?(x=w488) -> (x >= 0?=w486:bool[])
        n310 = And Array Elements(Boolean array=w486) -> ()  [unwired: 1 out]
        n311 = Index Array(array=w487, index #1=0 ("index"), index #2=1 ("index"), index #3=2 ("index")) -> (element #1=w479:i32, element #2=w480:i32, element #3=w481:i32)
        n312 = Multiply(x=w480, y=w478) -> (x*y=w476:dbl)
        n313 = Multiply(x=w481, y=w478) -> (x*y=w475:dbl)
        n314 = Multiply(x=w479, y=w478) -> (x*y=w477:dbl)
        n315 = local write "Destination Y"(w475) -> ()
        n316 = local write "Destination Z"(w477) -> ()
        n317 = local write "Destination X"(w476) -> ()
      }
      frame "Copy Positions" {
        # "When \"Copy Positions\" button is pressed, the current cursor values will be copied to the Clipboad. These values can then be pasted in an Excel file."
        n318 = property on="Cursor Z" class="DigNum (strict)"() -> ("Value"=w496:dbl)  [unwired: 2 in, 2 out]
        n319 = property on="Cursor X" class="DigNum (strict)"() -> ("Value"=w498:dbl)  [unwired: 2 in, 2 out]
        n320 = property on="Cursor Y" class="DigNum (strict)"() -> ("Value"=w497:dbl)  [unwired: 2 in, 2 out]
        n321 = Build Array(w498, w497, w496) -> (w499:dbl[])
        n322 = Array To Spreadsheet String(array=w499, 3:"%.3f" ("initial string")) -> (spreadsheet string=w503:string)  [unwired: 1 in]
        n323 = invoke class="App" method="Clipboard.Write"("Param 0"=w503) -> ()  [unwired: 3 in, 4 out]
      }
      frame "Paste Positions" {
        # "When \"Paste Positions\" button is pressed, the  values stored in the Clipboard will be pasted in the \"Move to Destination\" inputs."
        n324 = invoke class="App" method="Clipboard.Read"() -> ("Read Clipbrd"=w511:string)  [unwired: 3 in, 2 out]
        n325 = Spreadsheet String To Array(format string="", spreadsheet string=w511, array type (2D Dbl)=dbl[] [] ("Array")) -> (array=w508:dbl[])  [unwired: 1 in]
        n326 = Index Array(array=w508) -> (element #1=w507:dbl, element #2=w506:dbl, element #3=w505:dbl)  [unwired: 3 in]
        n327 = property on="Destination X" class="DigNum (strict)"("Value"=w507) -> ()  [unwired: 2 in, 2 out]
        n328 = property on="Destination Z" class="DigNum (strict)"("Value"=w505) -> ()  [unwired: 2 in, 2 out]
        n329 = property on="Destination Y" class="DigNum (strict)"("Value"=w506) -> ()  [unwired: 2 in, 2 out]
      }
      frame "Exit" {
        n330 = Unbundle By Name(w522) -> ("IDs"=w524:i32[])
        n331 = for {
          tunnel: w524 -> [w525] mode=indexing
          n332 = call "close device.vi"("id"=w525) -> ()  [unwired: 8 in, 3 out]
        }
        n333 = Open Application Reference(8:errorcluster {"status"=FALSE, "code"=0, "source"=""} ("error in (no error)")) -> (0:w515:errorcluster, 3:w516:refnum<vi>)  [unwired: 3 in]
        n334 = property class="App"(reference=w516, error in=w515) -> ("App.Kind"=w519:T3)  [unwired: 2 out]
        n335 = Equal?(x=w519, y=T3."Run Time System" ("Application:Kind")) -> (x = y?=w517:bool)
        n336 = Quit LabVIEW(quit? (T)=w517) -> ()
      }
    }
  }
